vi "Filter Paths if Folder matches Pattern.vi"(6 "REP ( ^[_.] as Default)\nempty to disable this feature":string="^[_.]", 7 "Root Dir":path=path "C:/", 8 "error in (no error)":errorcluster, 11 "Paths":path[](array[path])) -> (0 "error in (no error) (dup)":errorcluster, 3 "Filted Paths":path[](array[path]))   [LabVIEW 2017]
uses:
  <userlib>/_OpenG.lib/file/file.llb/Compare Two Paths - Scalar__ogtk.vi
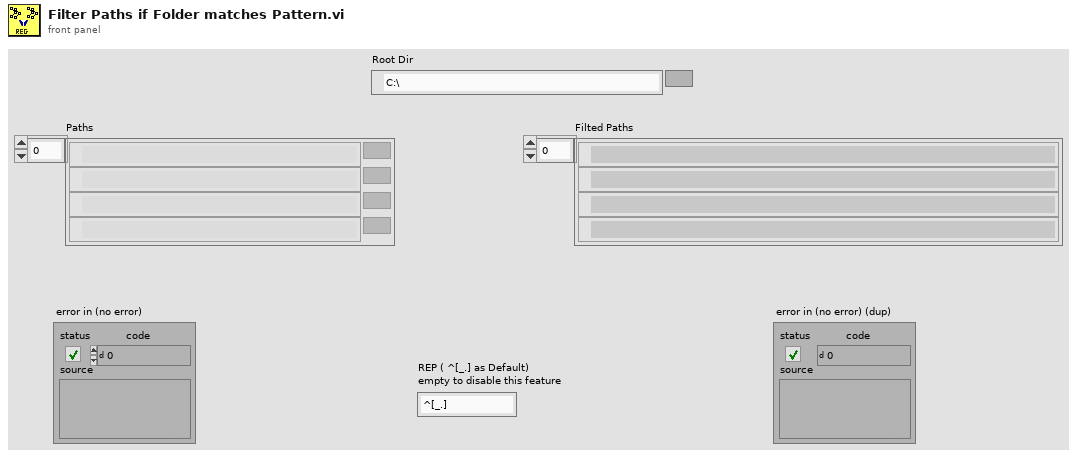
[diagram p1: front panel]
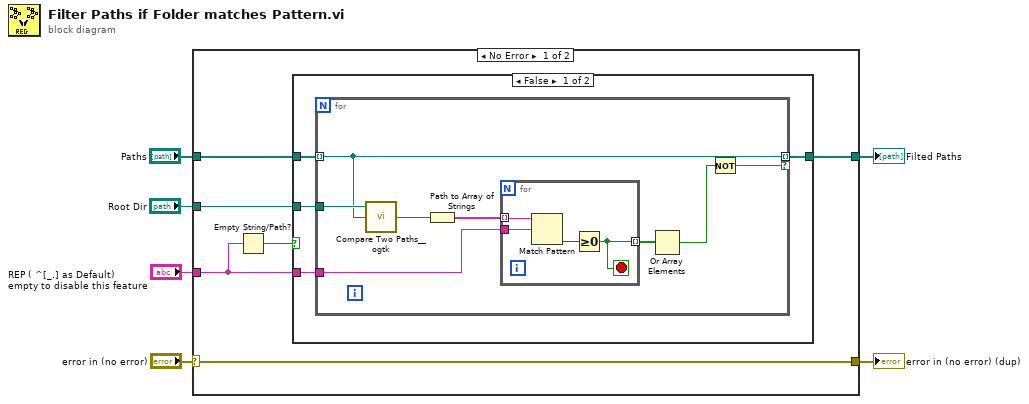
[diagram p0: block diagram]
diagram:
  n1 = case shown="No Error" "error in (no error)" {
    selector: "error in (no error)" -> [w9 w31]
    tunnel: "Paths" -> [w12 w30]
    tunnel: "Root Dir" -> [w11 _]
    tunnel: "REP ( ^[_.] as Default)\nempty to disable this feature" -> [w8 _]
    tunnel: [w10 w30] -> w3
    tunnel: [w9 w31] -> w1
    frame No Error {
      n2 = Empty String/Path?(string/path=w8) -> (empty?=w7:bool)
      n3 = case shown="False" w7 {
        tunnel: w12 -> [w16 w29]
        tunnel: w11 -> [w15 _]
        tunnel: [w14 w29] -> w10
        tunnel: w8 -> [w13 _]
        frame False {
          n4 = for {
            tunnel: w16 -> [w19] mode=indexing
            tunnel: w15 -> [w24]
            tunnel: w13 -> [w21]
            tunnel: [w19] -> w14 mode=indexing if=w17
            n5 = call-poly <userlib>:"Compare Two Paths__ogtk.vi"("path2"=w19, "path1"=w24) -> ("relative path from 1 to 2"=w23:path)  [unwired: 1 in, 2 out]
            n6 = Path to Array of Strings(0:w23) -> (2:w22:string[])  [unwired: 1 out]
            n7 = for {
              tunnel: w22 -> [w28] mode=indexing
              tunnel: w21 -> [w27]
              tunnel: [w25] -> w20 mode=indexing
              stop <- w25 stop-if-true
              n8 = Match Pattern(string=w28, regular expression=w27) -> (offset past match=w26:i32)  [unwired: 1 in, 3 out]
              n9 = Greater Or Equal To 0?(x=w26) -> (x >= 0?=w25:bool)
            }
            n10 = Or Array Elements(Boolean array=w20) -> (logical OR=w18:bool)
            n11 = Not(x=w18) -> (.not. x?=w17:bool)
          }
        }
        frame True {
        }
      }
    }
    frame Error {
    }
  }
  "Filted Paths" <- w3
  "error in (no error) (dup)" <- w1
